vi "Trav_Pos_Error.vi"(1 "Read Positions":dbl[](array[numeric]), 2 "GoTo Array":T1[](array[typedef]) {"Go To Position" step=100000.0}, 3 "Error strings":string[](array[string])) -> (0 "Error String":string)   [LabVIEW 2010]
uses:
  X-_Channel_Config_Global.vi
  X-_Ch_cluster.ctl
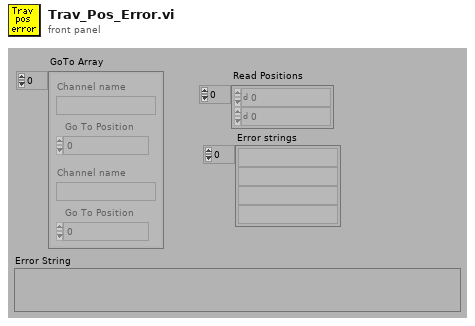
[diagram p1: front panel]
types:
  T1 = typedef "X-_Ch_cluster.ctl" = cluster{"Channel name":string, "Go To Position":dbl}
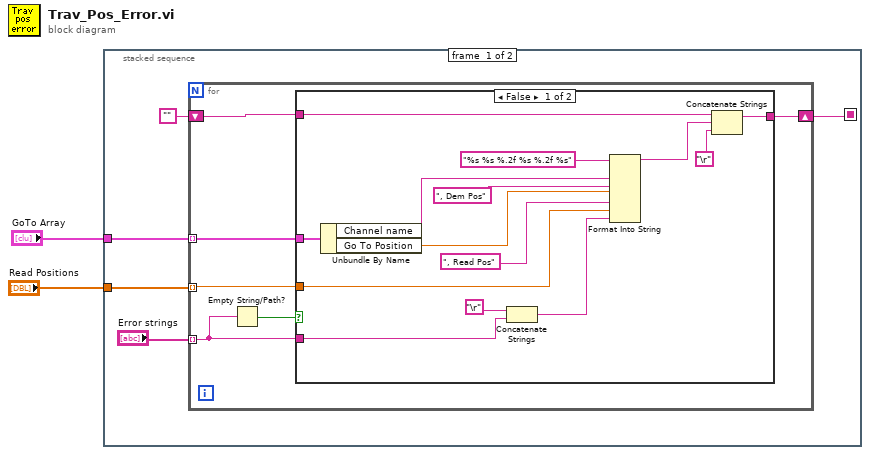
[diagram p0: block diagram]
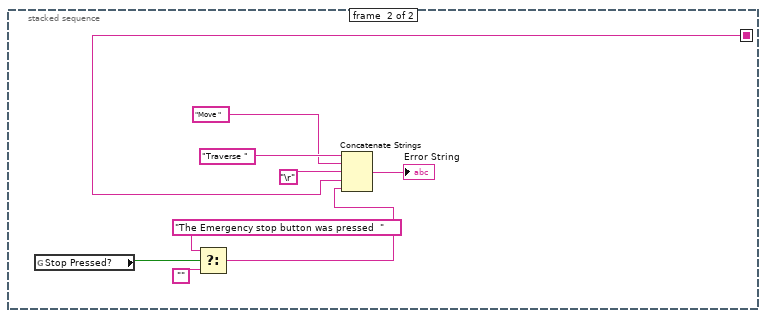
[diagram p3: hidden frame]
diagram:
  n1 = stacked-sequence {
    seq-local: [w3 _] -> [_ w34]
    tunnel: "Read Positions" -> [w7 _]
    tunnel: "GoTo Array" -> [w6 _]
    frame #0 {
      n2 = for {
        tunnel: w6 -> [w13] mode=indexing
        tunnel: w7 -> [w12] mode=indexing
        shift-right: [w10] -> w3
        shift-left: "" -> [w11]
        tunnel: "Error strings" -> [w9] mode=indexing
        n3 = Empty String/Path?(string/path=w9) -> (empty?=w8:bool)
        n4 = case shown="False" w8 {
          tunnel: w13 -> [w27 _]
          tunnel: w12 -> [w24 _]
          tunnel: w11 -> [w23 w28]
          tunnel: [w21 w28] -> w10
          tunnel: w9 -> [w14 _]
          frame False {
            n5 = Unbundle By Name(w27) -> ("Channel name"=w26:string, "Go To Position"=w25:dbl)
            n6 = Concatenate Strings("\r", w14) -> (w15:string)
            n7 = Format Into String(format string="%s %s %.2f %s %.2f %s", w26, ", Dem Pos", w25, ", Read Pos", w24, w15) -> (resulting string=w22:string)  [unwired: 2 in, 1 out]
            n8 = Concatenate Strings(w23, w22, "\r") -> (w21:string)
          }
          frame True {
          }
        }
      }
    }
    frame #1 {
      n9 = global read "X-_Channel_Config_Global.vi" "Stop Pressed?"() -> (w33:bool)
      n10 = Select(t="The Emergency stop button was pressed  ", s=w33, f="") -> (s? t:f=w30:string)
      n11 = Concatenate Strings("Traverse " ("source"), "Move ", "\r", w34, w30) -> (→"Error String":string)
    }
  }
